vi "Exemple_Metrics_Homogeneity_Score.vi"() -> ()   [LabVIEW 2020]
uses:
  Objet/3 - Model selection and evaluation/3.3 - Metrics and scoring/homogeneity_score/Homogeneity_Score.vi
panel:
  out "Score":string
  out "error out":errorcluster caption="sortie d'erreur"
  in  "error in (no error)":errorcluster caption="entrée d'erreur (pas d'erreur)"
  in  "labels_pred":string[][](array[string])=[["1"], ["1"], ["0"], ["0"]]
  in  "labels_true":string[][](array[string])=[["0"], ["0"], ["1"], ["1"]]
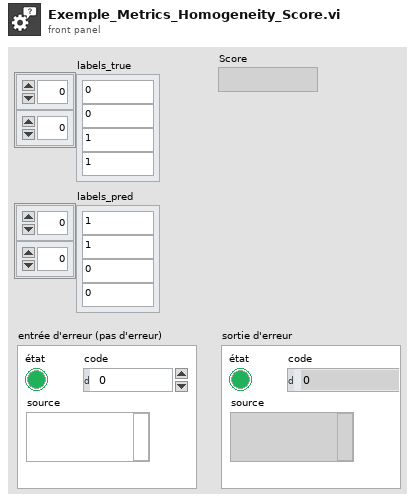
[diagram p1: front panel]
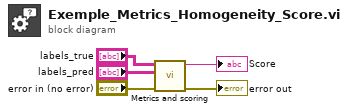
[diagram p0: block diagram]
diagram:
  n1 = call-poly "Metrics and scoring.vi"("error in (no error)"="error in (no error)", "labels_pred"="labels_pred", "labels_true"="labels_true") -> ("error out"=→"error out":errorcluster, "Score"=→"Score":string)  [unwired: 7 in]
